vi "Temperature Limit.vi"() -> ()   [LabVIEW 2012]
doc: "This VI simulates the acquisition of temperature, graphs the temperature, and notifies the user if the temperature is over the limit."
panel:
  in  "Start":bool
  in  "Delta t (ms)":i32(slide)=400 scale=50.0..500.0
  in  "Stop":bool
  in  "High Limit":dbl=28.0 format="%.2f"
  out "Temperature":cluster{"Temperature":dbl, "High Limit":dbl}(graph)={"Temperature"=85.88749999999999, "High Limit"=80.0}
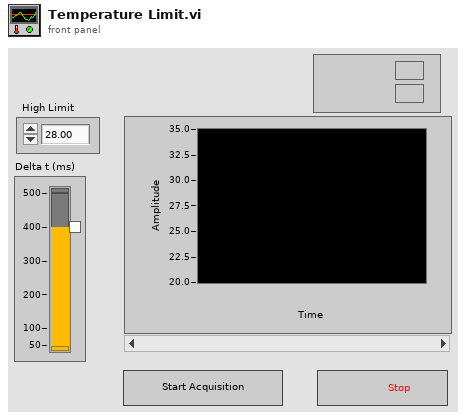
[diagram p1: front panel]
types:
  T1 = cluster{"Temperature Value":dbl, "High Limit":dbl}
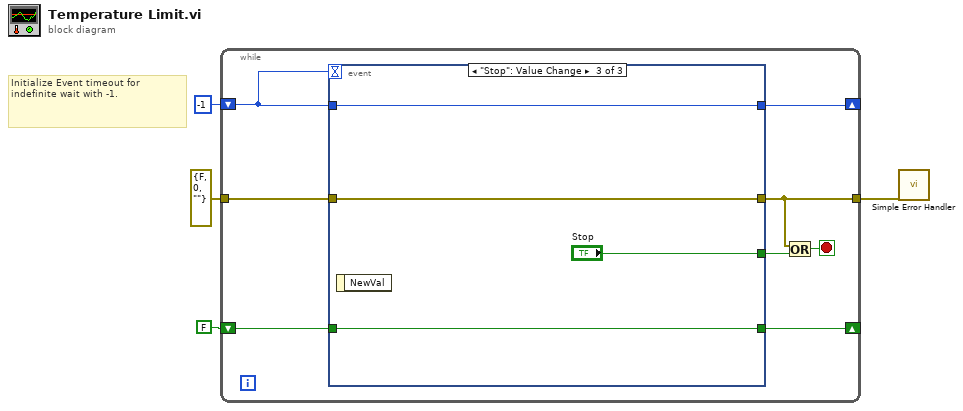
[diagram p0: block diagram]
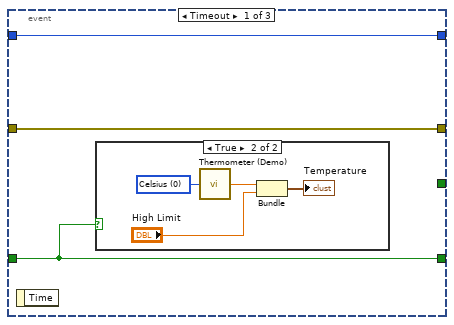
[diagram p2: hidden frame]
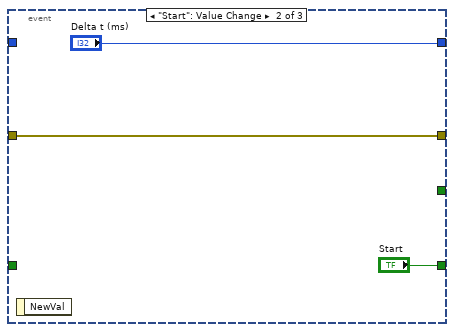
[diagram p4: hidden frame]
diagram:
  # "Initialize Event timeout for indefinite wait with -1."
  n1 = while {
    tunnel: errorcluster {"status"=FALSE, "code"=0, "source"=""} ("error out") -> [w12]
    tunnel: [w10] -> w3
    shift-right: [w8] -> _
    shift-left: FALSE ("Start") -> [w7]
    shift-right: [w6] -> _
    shift-left: -1 ("Delta t (ms)") -> [w5]
    stop <- w11 stop-if-true
    n2 = event shown="[2] \"Stop\": Value Change" {
      selector: _ -> [_ _ _]
      dyn-events: _ -> [_ _ _]
      timeout: w5 -> [_ _ _]
      tunnel: [_ _ "Stop"] -> w9
      tunnel: w12 -> [w15 w20 w25]
      tunnel: [w15 w20 w25] -> w10
      tunnel: [w13 "Start" w24] -> w8
      tunnel: w7 -> [w13 _ w24]
      tunnel: [w14 "Delta t (ms)" w23] -> w6
      tunnel: w5 -> [w14 _ w23]
      event Timeout {
        n3 = event-data() -> ()  [unwired: 1 in, 1 out]
        n4 = case shown="True" w13 {
          frame False {
          }
          frame True {
            w16 = u16 0 items=["Celsius", "Fahrenheit"] ("Units (0: Celsius)")
            n5 = call "Thermometer (Demo).vi"("Units (0: Celsius)"=w16) -> ("Temperature Value"=w17:dbl)
            n6 = Bundle("Temperature Value"=w17, "High Limit"="High Limit") -> (→"Temperature":T1)  [unwired: 1 in]
          }
        }
      }
      event "Start": Value Change {
        n7 = event-data() -> ()  [unwired: 1 in, 1 out]
      }
      event "Stop": Value Change {
        n8 = event-data() -> ()  [unwired: 1 in, 1 out]
      }
    }
    n9 = Or(x=w10, y=w9) -> (x .or. y?=w11:bool)
  }
  n10 = call <vilib>:"Simple Error Handler.vi"("error in (no error)"=w3) -> ()  [unwired: 4 in, 5 out]
